vi "Memory.Pointer.New.2B.vi"(8 "error in (no error)":errorcluster, 10 "count (1)":u64=1, 11 "pointer type":refnum<class "Memory.Pointer.lvclass">) -> (0 "error out":errorcluster, 3 "pointer out":refnum<class "Memory.Pointer.lvclass">)   [LabVIEW 2016, in "Memory.lvlib" / "Memory.Pointer.lvclass"]
uses:
  Memory.Pointer.lvclass
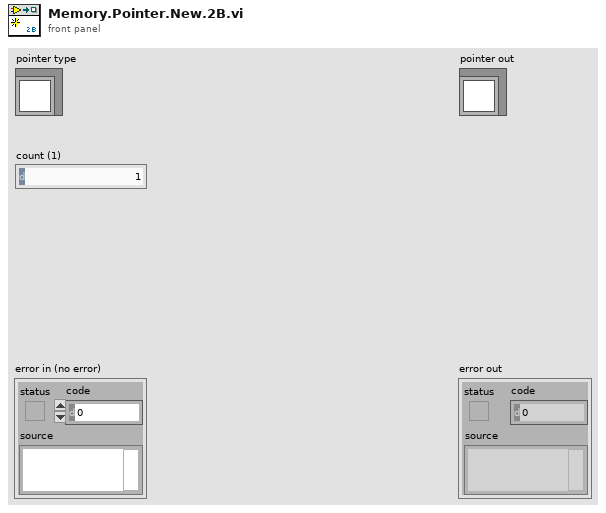
[diagram p1: front panel]
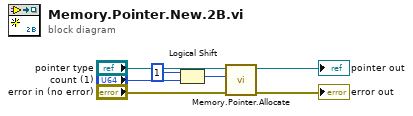
[diagram p0: block diagram]
diagram:
  n1 = Logical Shift(y=i16 1, x="count (1)") -> (x << y=w2:u64)
  n2 = call "Memory.Pointer.Allocate.vi"("error in (no error)"="error in (no error)", "size"=w2, "pointer in"="pointer type") -> ("error out"=→"error out":errorcluster, "pointer out"=→"pointer out":refnum<class "Memory.Pointer.lvclass">)  [unwired: 7 in]
